vi "sppf single step from kalman.vi"(10 "kalman result":T2, 11 "SPPF state":T1={"theta"=[0.0, 0.0], "w"=[[1000000000.0, 0.0], [0.0, 100000000.0]], "elapsed time"=0.0}) -> (0 "ratio":dbl, 1 "green rate":dbl, 2 "red rate":dbl, 3 "SPPF state out":T1, 4 "green rate direct":dbl, 5 "theta out":dbl[](array[numeric]), 6 "red rate direct":dbl)   [LabVIEW 2010]
uses:
  kalman_result_scaled.ctl
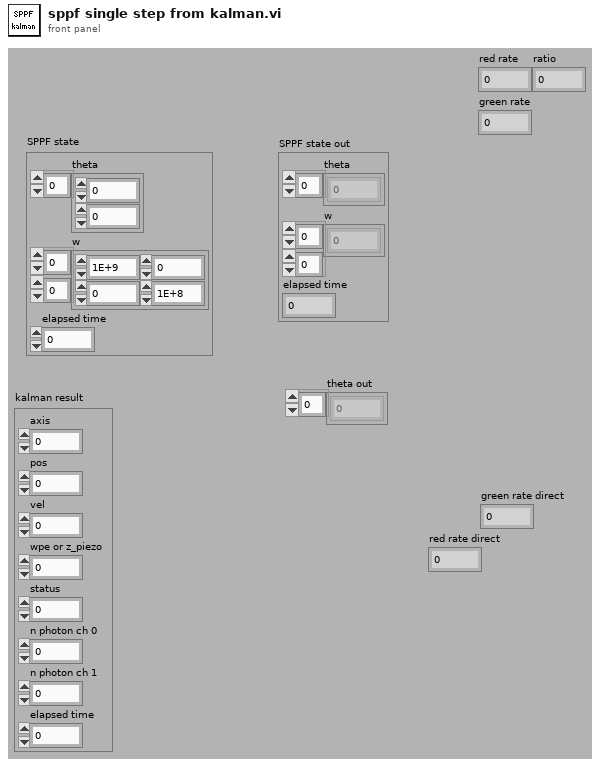
[diagram p1: front panel]
types:
  T1 = cluster{"theta":dbl[], "w":dbl[][], "elapsed time":dbl}
  T2 = typedef "kalman_result_scaled.ctl" = cluster{"axis":u8, "pos":dbl, "vel":dbl, "wpe or z_piezo":dbl, "status":u32, "n photon ch 0":u32, "n photon ch 1":u32, "elapsed time":dbl}
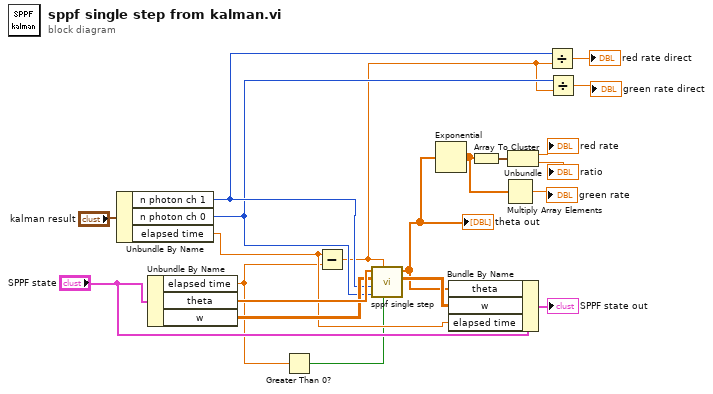
[diagram p0: block diagram]
diagram:
  n1 = Unbundle By Name("kalman result") -> ("n photon ch 1"=w7:u32, "n photon ch 0"=w5:u32, "elapsed time"=w16:dbl)
  n2 = Unbundle By Name("SPPF state") -> ("elapsed time"=w2:dbl, "theta"=w19:dbl[], "w"=w18:dbl[][])
  n3 = Greater Than 0?(x=w2) -> (x > 0?=w1:bool)
  n4 = Subtract(x=w16, y=w2) -> (x-y=w4:dbl)
  n5 = call "sppf single step.vi"("do update"=w1, "dt"=w4, "num green photons"=w5, "num red photons"=w7, "w"=w18, "theta"=w19) -> ("w"=w17:dbl[][], "theta"=w13:dbl[])  [unwired: 3 in, 1 out]
  "theta out" <- w13
  n6 = Exponential(1:w13) -> (0:w9:dbl[])
  n7 = Bundle By Name(cluster="SPPF state", "theta"=w13, "w"=w17, "elapsed time"=w16) -> (→"SPPF state out":T1)
  n8 = Array To Cluster(array=w9) -> (cluster=w12:cluster{"[0]":dbl, "[1]":dbl})
  n9 = Multiply Array Elements(1:w9) -> (0:→"green rate":dbl)
  n10 = Unbundle(w12) -> ("[0]"=→"red rate":dbl, "[1]"=→"ratio":dbl)
  n11 = Divide(x=w7, y=w4) -> (x/y=→"red rate direct":dbl)
  n12 = Divide(x=w5, y=w4) -> (x/y=→"green rate direct":dbl)
